vi "update setup complete.vi"() -> ()   [LabVIEW 2014]
panel:
  in  "?":bool
  out "?":string
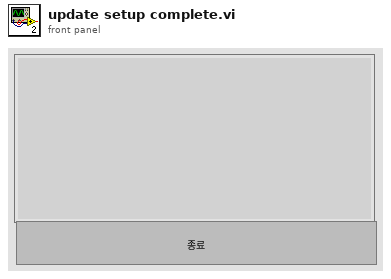
[diagram p1: front panel]
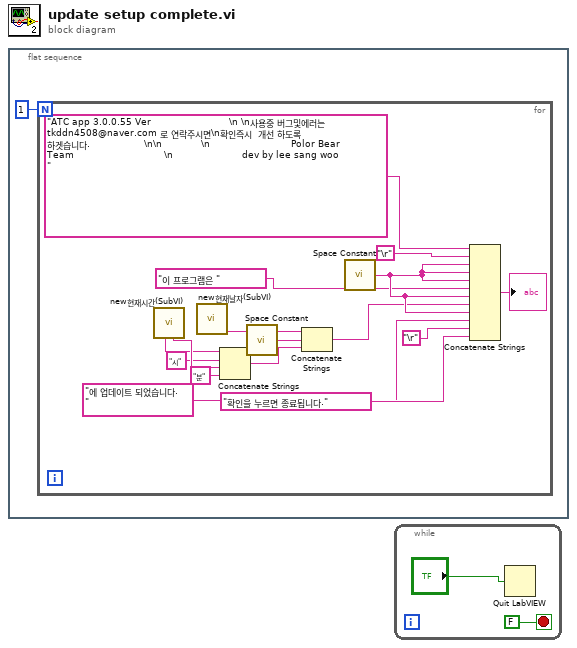
[diagram p0: block diagram]
diagram:
  n1 = flat-sequence {
    frame #0 {
      n2 = for {
        N: 1 -> [_]
        n3 = call "new현재시간(SubVI).vi"() -> ("분 문자열"=w4:string, "시 문자열"=w2:string)  [unwired: 3 in, 7 out]
        n4 = call "new현재날자(SubVI).vi"() -> ("월,일 을 문자열로"=w8:string)  [unwired: 5 in, 6 out]
        n5 = Concatenate Strings(w2, "시", w4, "분" ("문자열")) -> (w6:string)
        n6 = call <vilib>:"Space Constant.vi"() -> ("String"=w7:string)
        n7 = Concatenate Strings(w8, w7, w6) -> (w12:string)
        n8 = call <vilib>:"Space Constant.vi"() -> ("String"=w13:string)
        n9 = Concatenate Strings("ATC app 3.0.0.55 Ver                          \n \n사용중 버그및에러는 tkddn4508@naver.com 로 연락주시면\n확인즉시  개선 하도록 하겟습니다.                  \n\n             \n                           Polor Bear Team                              \n                       dev by lee sang woo                            " ("Message"), "\r", w13, w13, w13, "이 프로그램은 ", w13, w12, w13, "에 업데이트 되었습니다.", "\r", "확인을 누르면 종료됩니다.") -> (→"?":string)
      }
    }
  }
  n10 = while {
    stop <- FALSE stop-if-true
    n11 = Quit LabVIEW(quit? (T)="?") -> ()
  }
